vi "Value By Name.vi"(7 "Column Type":refnum<class "Type.lvclass">, 10 "Name":string, 11 "Result Row in":refnum<class "Result Row.lvclass">) -> (0 "error out":errorcluster, 2 "Value":refnum<class "Type.lvclass">)   [LabVIEW 2020, in "Conditum.lvlib" / "Result Row.lvclass"]
uses:
  Result Row.lvclass
  Columns/Type/Type.lvclass
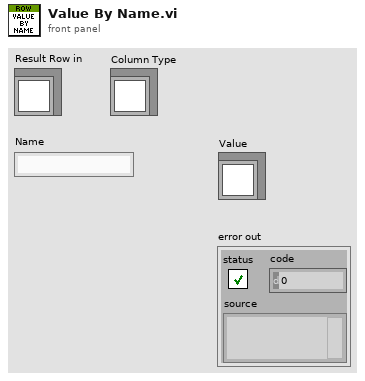
[diagram p1: front panel]
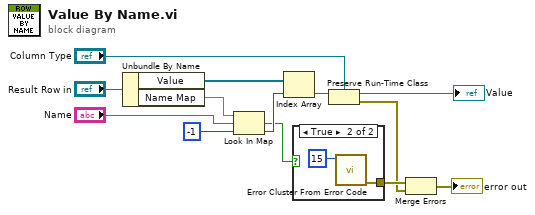
[diagram p0: block diagram]
diagram:
  n1 = Unbundle By Name("Result Row in") -> ("Value"=w9:refnum<class "Type.lvclass">[], "Name Map"=w12:map{string, i32})
  n2 = Look In Map(map=w12, key="Name", default value=-1) -> (key not found?=w4:bool, value=w8:i32)
  n3 = Index Array(array=w9, index=w8) -> (element=w7:refnum<class "Type.lvclass">)
  n4 = case shown="True" w4 {
    tunnel: [_ w14] -> w3
    frame False {
    }
    frame True {
      n5 = call <vilib>:"Error Cluster From Error Code.vi"("error code (0)"=15) -> ("error out"=w14:errorcluster)  [unwired: 8 in]
    }
  }
  n6 = Preserve Run-Time Class(object in=w7, 2:"Column Type") -> (object out=→"Value":refnum<class "Type.lvclass">, error out=w2:errorcluster)  [unwired: 1 in]
  n7 = Merge Errors(w3, w2) -> (→"error out":errorcluster)
